vi "Compile Battery Switch.vi"(8 "error in (no error)":errorcluster, 11 "Device Item Ref in":T5 format="%.0x") -> (0 "error out":errorcluster, 1 "Battery Switch Engine Data":T1 {"Ordered Channels" format="%.0x"; "RT IDs"."Slot #" max=15; "RT IDs"."Chip Address (A2 A1 A0)" max=7}, 2 "Initial Battery Switch SPI CMDs":u64[](array[numeric]), 3 "Device Item Ref out":T5 format="%.0x")   [LabVIEW 2014, in "SLSC configuration System Explorer.lvlib"]
uses:
  SLSC configuration System Explorer.lvlib
  <vilib>/NI Veristand/Custom Device API/Custom Device Item Ref.ctl
  Shared/Type Defs/RT Engine Data.ctl
  Shared/Type Defs/RT IDs.ctl
  Shared/SPI Utility/Slot #.ctl
  Shared/MCP23S17/Chip Address.ctl
  Shared/Constants.vi
  <vilib>/NI Veristand/Custom Device Tools/Custom Device Utility Library/Custom Device Utility Library.lvlib
  Shared/SLSC configuration Shared.lvlib
  <vilib>/NI Veristand/Custom Device API/Custom Device API.lvlib
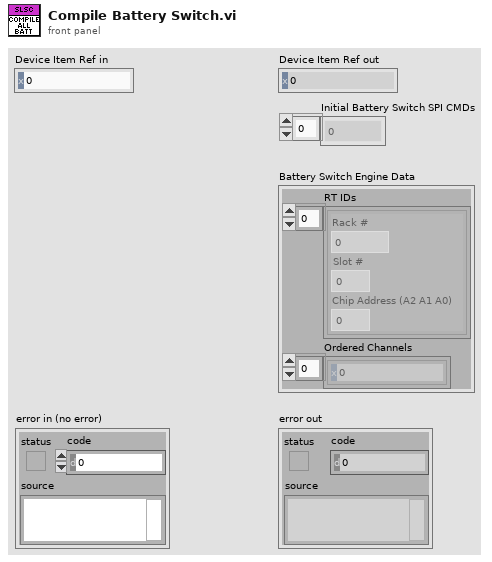
[diagram p1: front panel]
types:
  T1 = typedef "SLSC configuration Shared.lvlib/RT Engine Data.ctl" = cluster{"RT IDs":T2[], "Ordered Channels":T5[]}
  T2 = typedef "SLSC configuration Shared.lvlib/RT IDs.ctl" = cluster{"Rack #":u8, "Slot #":T3, "Chip Address (A2 A1 A0)":T4}
  T3 = typedef "SLSC configuration Shared.lvlib/Slot #.ctl" = u8
  T4 = typedef "SLSC configuration Shared.lvlib/Chip Address.ctl" = u8
  T5 = typedef "Custom Device API.lvlib/Custom Device Item Ref.ctl" = u64
  T6 = typedef "SLSC configuration Shared.lvlib/Card Position.ctl" = cluster{"Rack #":u8, "Slot #":T3}
  T7 = typedef "SLSC configuration Shared.lvlib/Battery Switch.ctl" = enum8{"Off", "On"}
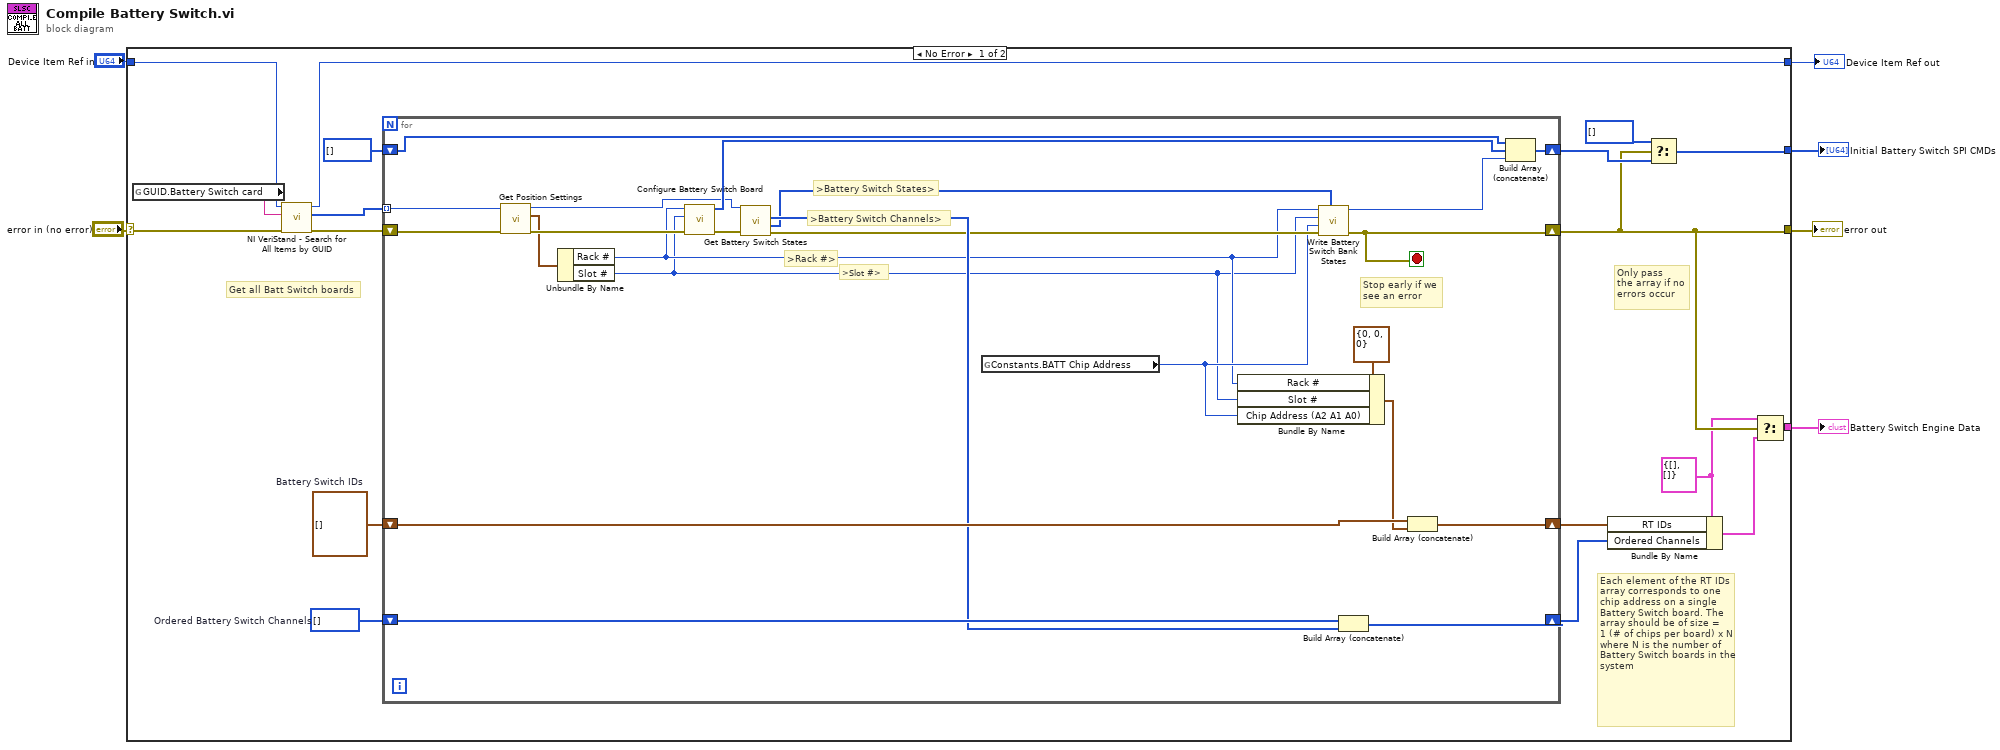
[diagram p0: block diagram]
diagram:
  n1 = case shown="No Error" "error in (no error)" {
    selector: "error in (no error)" -> [w21 w49]
    tunnel: [w10 w49] -> w6
    tunnel: "Device Item Ref in" -> [w15 w48]
    tunnel: [w7 _] -> w3
    tunnel: [w11 _] -> w2
    tunnel: [w14 w48] -> w1
    frame No Error {
      w9 = T1 {"RT IDs"=[], "Ordered Channels"=[]} ("FIU Engine Data")
      w18 = T5[] []  # Ordered Battery Switch Channels
      w19 = T2[] []  # Battery Switch IDs
      # "Only pass\nthe array if no\nerrors occur"
      # "Get all Batt Switch boards"
      # "Each element of the RT IDs array corresponds to one chip address on a single Battery Switch board. The array should be of size =\n1 (# of chips per board) x N where N is the number of Battery Switch boards in the system"
      n2 = global read "Constants.vi" "GUID.Battery Switch card"() -> (w24:string)
      n3 = call <vilib>:"NI VeriStand - Search for All Items by GUID.vi"("error in"=w21, "Item GUID"=w24, "Section Ref in"=w15) -> ("error out"=w23:errorcluster, "Item Refs"=w22:T5[], "Section Ref out"=w14:T5)  [unwired: 5 in, 1 out]
      n4 = for {
        tunnel: w22 -> [w31] mode=indexing
        shift-right: [w36] -> w10
        shift-left: w23 -> [w30]
        shift-right: [w43] -> w13
        shift-left: u64[] [] ("SPI FIFO Messages") -> [w47]
        shift-right: [w41] -> w17
        shift-left: w19 -> [w42]
        shift-right: [w39] -> w16
        shift-left: w18 -> [w40]
        stop <- w36 stop-if-true
        # ">Battery Switch States>"
        # "Stop early if we\nsee an error"
        # ">Battery Switch Channels>"
        # ">Slot #>"
        # ">Rack #>"
        n5 = call "Get Position Settings.vi"("error in (no error)"=w30, "Item Ref in"=w31) -> ("error out"=w29:errorcluster, "Card Position"=w27:T6, "Item Ref out"=w28:T5)  [unwired: 7 in]
        n6 = Unbundle By Name(w27) -> ("Rack #"=w26:u8, "Slot #"=w25:T3)
        n7 = call "Configure Battery Switch Board.vi"("error in (no error)"=w29, "Slot #"=w25, "Rack #"=w26) -> ("error out"=w45:errorcluster, "SPI FIFO Messages"=w46:u64[])  [unwired: 7 in]
        n8 = call "Get Battery Switch States.vi"("error in (no error)"=w45, "Item Ref in"=w28) -> ("error out"=w37:errorcluster, "Battery Switch States"=w34:T7[], "Ordered Battery Switch Channels"=w38:T5[])  [unwired: 6 in, 1 out]
        n9 = global read "Constants.vi" "Constants.BATT Chip Address"() -> (w35:u8)
        n10 = Bundle By Name(cluster=T2 {"Rack #"=0, "Slot #"=0, "Chip Address (A2 A1 A0)"=0}, "Rack #"=w26, "Slot #"=w25, "Chip Address (A2 A1 A0)"=w35) -> (w32:T2)
        n11 = call "Write Battery Switch Bank States.vi"("Battery Switch States"=w34, "error in (no error)"=w37, "Chip Address (A2 A1 A0)"=w35, "Slot #"=w25, "Rack #"=w26) -> ("error out"=w36:errorcluster, "FIFO SPI Message"=w44:u64)  [unwired: 4 in, 1 out]
        n12 = Build Array (concatenate)(w40, w38) -> (w39:T5[])
        n13 = Build Array (concatenate)(w42, w32) -> (w41:T2[])
        n14 = Build Array (concatenate)(w47, w46, w44) -> (w43:u64[])
      }
      n15 = Bundle By Name(cluster=w9, "RT IDs"=w17, "Ordered Channels"=w16) -> (w8:T1)
      n16 = Select(t=u64[] [], s=w10, f=w13) -> (s? t:f=w11:u64[])
      n17 = Select(t=w9, s=w10, f=w8) -> (s? t:f=w7:T1)
    }
    frame Error {
    }
  }
  "error out" <- w6
  "Device Item Ref out" <- w1
  "Battery Switch Engine Data" <- w3
  "Initial Battery Switch SPI CMDs" <- w2
